vi "WriteFlagImpairParamsRequest.vi"(8 "error in (no error)":errorcluster, 10 "dblFlagImpairParams":T1, 11 "ModuleID":i32=-1) -> (0 "error out":errorcluster)   [LabVIEW 2014, in "FlagImpairModule.lvlib"]
uses:
  FlagImpairModule.lvlib
  PublicAPI/Arguments/Requests/dblFlagImpairParams.ctl
  clEventType.ctl
  <vilib>/Utility/error.llb/Error Cluster From Error Code.vi
  <vilib>/ErrorRing/Error Ring.xnode
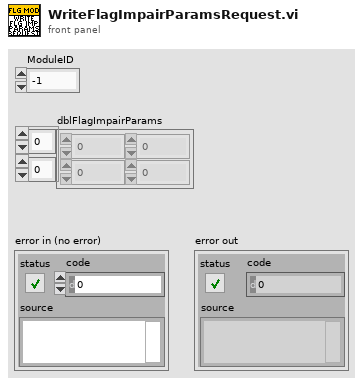
[diagram p1: front panel]
types:
  T1 = typedef "FlagImpairModule.lvlib/dblFlagImpairParams.ctl" = dbl[][]
  T2 = typedef "FlagImpairModule.lvlib/clRequestEvents.ctl" = cluster{"StopRequest":refnum<user-event>, "WriteFlagImpairConfigRequest":refnum<user-event>, "ReadFlagImpairConfigRequest":refnum<user-event>, "WriteFlagImpairParamsRequest":refnum<user-event>, "ReadFlagImpairParamsRequest":refnum<user-event>, "WriteTimeArrayRequest":refnum<user-event>, "ReadTimeArrayRequest":refnum<user-event>, "GetFlagImpairmentRequest":refnum<user-event>, "LoadPluginRequest":refnum<user-event>, "ReadPluginPathRequest":refnum<user-event>, "ShowPanelRequest":refnum<user-event>}
  T3 = typedef "FlagImpairModule.lvlib/clEventType.ctl" = cluster{"ModuleID":i32, "Data":variant}
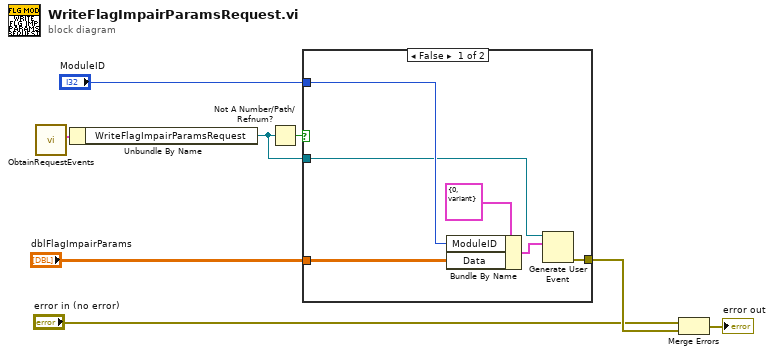
[diagram p0: block diagram]
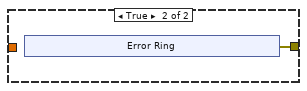
[diagram p2: hidden frame]
diagram:
  n1 = call "ObtainRequestEvents.vi"() -> ("clRequestEvents"=w8:T2)  [unwired: 10 in, 1 out]
  n2 = Unbundle By Name(w8) -> ("WriteFlagImpairParamsRequest"=w6:refnum<user-event>)
  n3 = Not A Number/Path/Refnum?(number/path/refnum=w6) -> (NaN/Path/Refnum?=w7:bool)
  n4 = case shown="False" w7 {
    tunnel: w6 -> [w12 _]
    tunnel: "dblFlagImpairParams" -> [w9 _]
    tunnel: "ModuleID" -> [w13 _]
    tunnel: [w10 w15] -> w2
    frame False {
      n5 = Bundle By Name(cluster=T3 {"ModuleID"=0, "Data"=variant} ("clEventType"), "ModuleID"=w13, "Data"=w9) -> (w11:T3)
      n6 = Generate User Event(user event=w12, event data cluster=w11) -> (error out=w10:errorcluster)  [unwired: 2 in, 1 out]
    }
    frame True {
      n7 = xnode "Error Ring"() -> ("error out"=w15:errorcluster)
    }
  }
  n8 = Merge Errors("error in (no error)", w2) -> (→"error out":errorcluster)
